vi "Zstd code to error.vi"() -> ()   [LabVIEW 2020, in "lvzstd.lvlib" / "lvzstd.lvclass"]
uses:
  lvzstd.lvclass
  <vilib>/Utility/error.llb/Error Cluster From Error Code.vi
  <vilib>/ErrorRing/Error Ring.xnode
  lvzstd.lvclass/lvzstd.ctl
panel:
  in  "Error code":i32
  out "error in (no error)":errorcluster
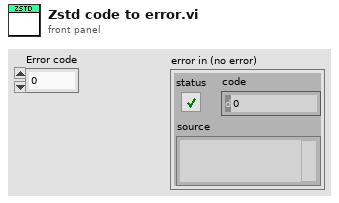
[diagram p1: front panel]
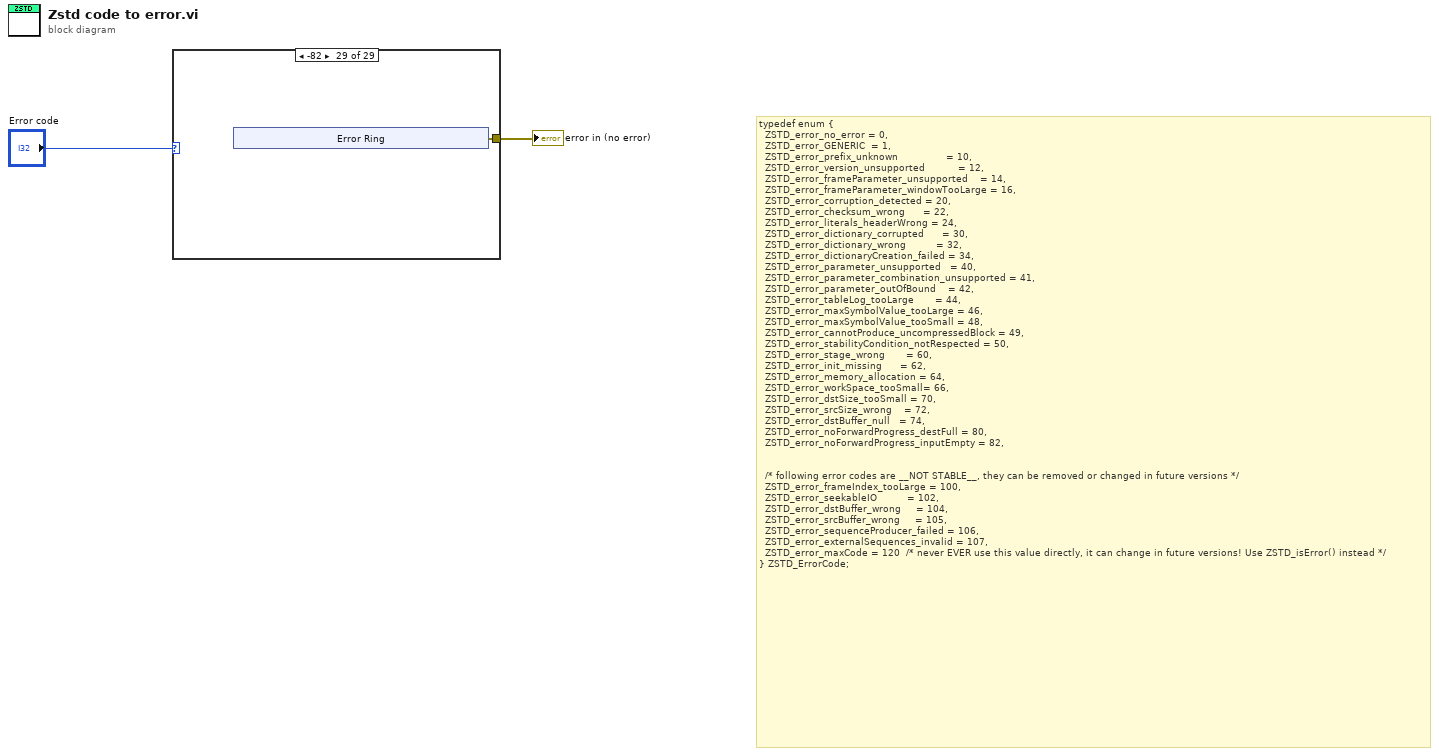
[diagram p0: block diagram]
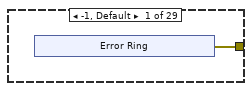
[diagram p2: hidden frame]
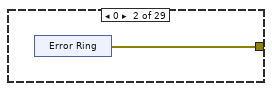
[diagram p3: hidden frame]
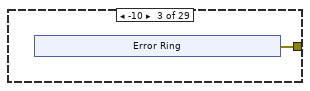
[diagram p4: hidden frame]
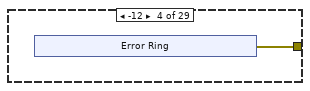
[diagram p5: hidden frame]
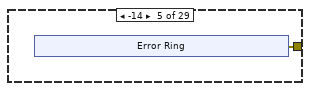
[diagram p6: hidden frame]
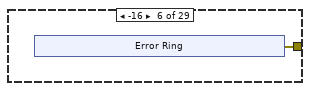
[diagram p7: hidden frame]
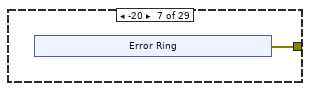
[diagram p8: hidden frame]
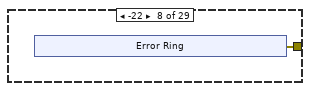
[diagram p9: hidden frame]
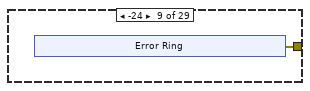
[diagram p10: hidden frame]
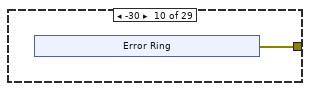
[diagram p11: hidden frame]
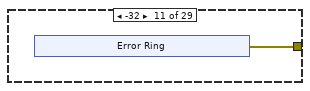
[diagram p12: hidden frame]
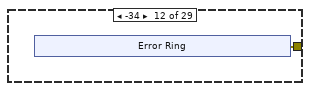
[diagram p13: hidden frame]
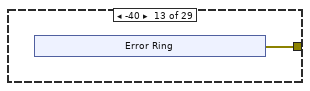
[diagram p14: hidden frame]
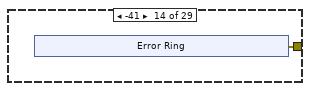
[diagram p15: hidden frame]
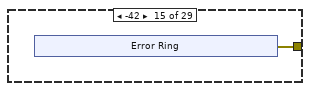
[diagram p16: hidden frame]
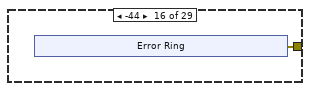
[diagram p17: hidden frame]
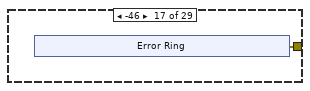
[diagram p18: hidden frame]
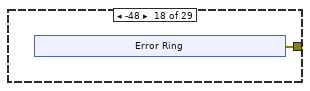
[diagram p19: hidden frame]
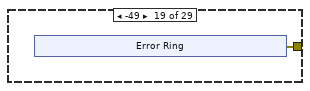
[diagram p20: hidden frame]
diagram:
  # "typedef enum {\n  ZSTD_error_no_error = 0,\n  ZSTD_error_GENERIC  = 1,\n  ZSTD_error_prefix_unknown                = 10,\n  ZSTD_error_version_unsupported           = 12,\n  ZSTD_error_frameParameter_unsupported    = 14,\n  ZSTD_error_frameParameter_windowTooLarge = 16,\n  ZSTD_error_corruption_detected = 20,\n  ZSTD_error_checksum_wrong      = 22,\n  ZSTD_error_literals_headerWrong = 24,\n  ZSTD_error_dictionary_corrupted      = 30,\n  ZSTD_error_dictionary_wrong          = 32,\n  ZSTD_error_dictionaryCreation_failed = 34,\n  ZSTD_error_parameter_unsupported   = 40,\n  ZSTD_error_parameter_combination_unsupported = 41,\n  ZSTD_error_parameter_outOfBound    = 42,\n  ZSTD_error_tableLog_tooLarge       = 44,\n  ZSTD_error_maxSymbolValue_tooLarge = 46,\n  ZSTD_error_maxSymbolValue_tooSmall = 48,\n  ZSTD_error_cannotProduce_uncompressedBlock = 49,\n  ZSTD_error_stabilityCondition_notRespected = 50,\n  ZSTD_error_stage_wrong       = 60,\n  ZSTD_error_init_missing      = 62,\n  ZSTD_error_memory_allocation = 64,\n  ZSTD_error_workSpace_tooSmall= 66,\n  ZSTD_error_dstSize_tooSmall = 70,\n  ZSTD_error_srcSize_wrong    = 72,\n  ZSTD_error_dstBuffer_null   = 74,\n  ZSTD_error_noForwardProgress_destFull = 80,\n  ZSTD_error_noForwardProgress_inputEmpty = 82,\n\n\n  /* following error codes are __NOT STABLE__, they can be removed or changed in future versions */\n  ZSTD_error_frameIndex_tooLarge = 100,\n  ZSTD_error_seekableIO          = 102,\n  ZSTD_error_dstBuffer_wrong     = 104,\n  ZSTD_error_srcBuffer_wrong     = 105,\n  ZSTD_error_sequenceProducer_failed = 106,\n  ZSTD_error_externalSequences_invalid = 107,\n  ZSTD_error_maxCode = 120  /* never EVER use this value directly, it can change in future versions! Use ZSTD_isError() instead */\n} ZSTD_ErrorCode;"
  n1 = case shown="-82" "Error code" {
    tunnel: [w3 w8 w10 w15 w20 w25 w30 w35 w40 w45 w50 w55 w60 w65 w70 w75 w80 w85 w90 w95 w100 w105 w110 w115 w120 w125 w130 w135 w140] -> w1
    frame -1, Default {
      n2 = xnode "Error Ring"() -> ("error out"=w3:errorcluster)
    }
    frame 0 {
      n3 = xnode "Error Ring"() -> ("error out"=w8:errorcluster)
    }
    frame -10 {
      n4 = xnode "Error Ring"() -> ("error out"=w10:errorcluster)
    }
    frame -12 {
      n5 = xnode "Error Ring"() -> ("error out"=w15:errorcluster)
    }
    frame -14 {
      n6 = xnode "Error Ring"() -> ("error out"=w20:errorcluster)
    }
    frame -16 {
      n7 = xnode "Error Ring"() -> ("error out"=w25:errorcluster)
    }
    frame -20 {
      n8 = xnode "Error Ring"() -> ("error out"=w30:errorcluster)
    }
    frame -22 {
      n9 = xnode "Error Ring"() -> ("error out"=w35:errorcluster)
    }
    frame -24 {
      n10 = xnode "Error Ring"() -> ("error out"=w40:errorcluster)
    }
    frame -30 {
      n11 = xnode "Error Ring"() -> ("error out"=w45:errorcluster)
    }
    frame -32 {
      n12 = xnode "Error Ring"() -> ("error out"=w50:errorcluster)
    }
    frame -34 {
      n13 = xnode "Error Ring"() -> ("error out"=w55:errorcluster)
    }
    frame -40 {
      n14 = xnode "Error Ring"() -> ("error out"=w60:errorcluster)
    }
    frame -41 {
      n15 = xnode "Error Ring"() -> ("error out"=w65:errorcluster)
    }
    frame -42 {
      n16 = xnode "Error Ring"() -> ("error out"=w70:errorcluster)
    }
    frame -44 {
      n17 = xnode "Error Ring"() -> ("error out"=w75:errorcluster)
    }
    frame -46 {
      n18 = xnode "Error Ring"() -> ("error out"=w80:errorcluster)
    }
    frame -48 {
      n19 = xnode "Error Ring"() -> ("error out"=w85:errorcluster)
    }
    frame -49 {
      n20 = xnode "Error Ring"() -> ("error out"=w90:errorcluster)
    }
    frame -50 {
      n21 = xnode "Error Ring"() -> ("error out"=w95:errorcluster)
    }
    frame -60 {
      n22 = xnode "Error Ring"() -> ("error out"=w100:errorcluster)
    }
    frame -62 {
      n23 = xnode "Error Ring"() -> ("error out"=w105:errorcluster)
    }
    frame -64 {
      n24 = xnode "Error Ring"() -> ("error out"=w110:errorcluster)
    }
    frame -66 {
      n25 = xnode "Error Ring"() -> ("error out"=w115:errorcluster)
    }
    frame -70 {
      n26 = xnode "Error Ring"() -> ("error out"=w120:errorcluster)
    }
    frame -72 {
      n27 = xnode "Error Ring"() -> ("error out"=w125:errorcluster)
    }
    frame -74 {
      n28 = xnode "Error Ring"() -> ("error out"=w130:errorcluster)
    }
    frame -80 {
      n29 = xnode "Error Ring"() -> ("error out"=w135:errorcluster)
    }
    frame -82 {
      n30 = xnode "Error Ring"() -> ("error out"=w140:errorcluster)
    }
  }
  "error in (no error)" <- w1
